vi "MACBIN Resource File Info Core__ogtk.vi"(5 "comment":string, 6 "error in (no error)":errorcluster, 7 "file info in":T1 {"mod date" format="%<%H:%M:%S\n%m/%d/%Y>T"; "creation date" format="%<%H:%M:%S\n%m/%d/%Y>T"}, 8 "write (F)":bool, 9 "resource file":path) -> (0 "error out":errorcluster, 1 "file info out":T1 {"mod date" format="%<%H:%M:%S\n%m/%d/%Y>T"; "creation date" format="%<%H:%M:%S\n%m/%d/%Y>T"}, 2 "is directory":bool, 3 "resource file out":path, 4 "comment out":string)   [LabVIEW 2014, in "ZLIB.lvlib"]
uses:
  ZLIB.lvlib
  MACBIN Resource Header__ogtk.ctl
  lvzlib.dll
panel:
  # "Please visit http://www.OpenG.org to learn about the\nOpen Source LabVIEW software movement.\n\nNOTICE -- YOU MUST LEAVE THIS NOTICE IN PLACE.  PER THE TERMS OF THE LICENSE BELOW, YOU MAY SUBLICENSE THIS SOFTWARE \nIN ANY WAY THAT DOES NOT CONFLICT WITH THIS LICENSE.\n\n### BSD License (http://www.opensource.org/licenses/bsd-license.php) Begin ###\n\nCopyright (C) 2006 Rolf Kalbermatter rolf.kalbermatter@citengineering.com\n\nAll rights reserved.\n\nRedistribution and use in source and binary forms, with or without modification, are permitted provided that the following conditions are met:\n\n    * Redistributions of source code must retain the above copyright notice, this list of conditions and the following disclaimer.\n    * Redistributions in binary form must reproduce the above copyright notice, this list of conditions and the following disclaimer in the \n       documentation and/or other materials provided with the distribution.\n    * Neither the name of SciWare, James Kring, Inc., nor the names of its contributors may be used to endorse or promote products derived \n       from this software without specific prior written permission.\n\nTHIS SOFTWARE IS PROVIDED BY THE COPYRIGHT HOLDERS AND CONTRIBUTORS \"AS IS\" AND ANY EXPRESS OR IMPLIED WARRANTIES, \nINCLUDING, BUT NOT LIMITED TO, THE IMPLIED WARRANTIES OF MERCHANTABILITY AND FITNESS FOR A PARTICULAR PURPOSE ARE \nDISCLAIMED. IN NO EVENT SHALL THE COPYRIGHT OWNER OR CONTRIBUTORS BE LIABLE FOR ANY DIRECT, INDIRECT, INCIDENTAL,\n SPECIAL, EXEMPLARY, OR CONSEQUENTIAL DAMAGES (INCLUDING, BUT NOT LIMITED TO, PROCUREMENT OF SUBSTITUTE GOODS OR \nSERVICES; LOSS OF USE, DATA, OR PROFITS; OR BUSINESS INTERRUPTION) HOWEVER CAUSED AND ON ANY THEORY OF LIABILITY, \nWHETHER IN CONTRACT, STRICT LIABILITY, OR TORT (INCLUDING NEGLIGENCE OR OTHERWISE) ARISING IN ANY WAY OUT OF THE USE \nOF THIS SOFTWARE, EVEN IF ADVISED OF THE POSSIBILITY OF SUCH DAMAGE.\n\n### BSD License End ###"
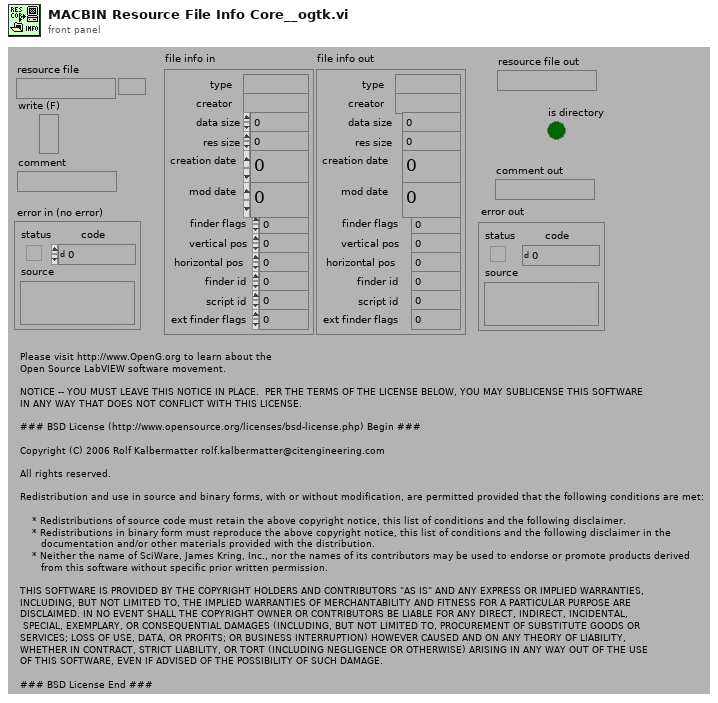
[diagram p1: front panel]
types:
  T1 = typedef "ZLIB.lvlib/MACBIN Resource Header__ogtk.ctl" = cluster{"type":string, "creator":string, "data size":u32, "res size":u32, "creation date":u32, "mod date":u32, "finder flags":u16, "vertical pos":i16, "horizontal pos":i16, "finder id":u16, "script id":u8, "ext finder flags":u8}
  T2 = cluster{"type":u32, "creator":u32, "data size":u32, "res size":u32, "creation date":u32, "mod date":u32, "finder flags":u16, "vertical pos":i16, "horizontal pos":i16, "finder id":u16, "script id":u8, "ext finder flags":u8}
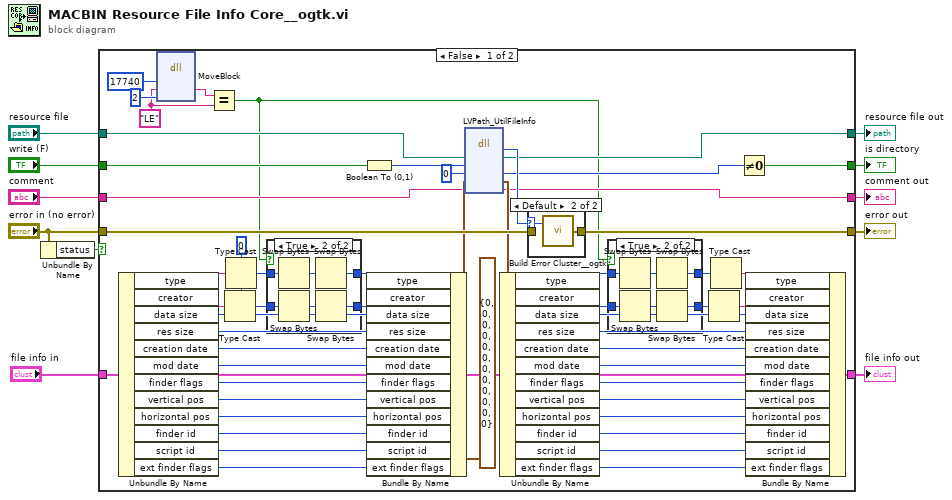
[diagram p0: block diagram]
diagram:
  n1 = Unbundle By Name("error in (no error)") -> ("status"=w2:bool)
  n2 = case shown="False" w2 {
    tunnel: [w27 w89] -> w7
    tunnel: "file info in" -> [w61 w90]
    tunnel: [w45 w90] -> w6
    tunnel: "comment" -> [w28 w89]
    tunnel: "write (F)" -> [w64 _]
    tunnel: [w65 w87] -> w9
    tunnel: "resource file" -> [w32 w88]
    tunnel: [w31 w88] -> w4
    tunnel: "error in (no error)" -> [w63 w87]
    tunnel: [w33 FALSE] -> w1
    frame False {
      w22 = "LE" ("y")
      w44 = u32 0 ("x")
      n3 = Unbundle By Name(w61) -> ("type"=w46:string, "creator"=w47:string, "data size"=w43:u32, "res size"=w42:u32, "creation date"=w41:u32, "mod date"=w40:u32, "finder flags"=w39:u16, "vertical pos"=w38:i16, "horizontal pos"=w37:i16, "finder id"=w36:u16, "script id"=w35:u8, "ext finder flags"=w34:u8)
      n4 = dll-call lib="LabVIEW" fn="MoveBlock"("src"=u16 17740, "dst"=w22, "len"=2) -> ("dst"=w21:string)  [unwired: 6 in, 2 out]
      n5 = Equal?(x=w21, y=w22) -> (x = y?=w12:bool)
      n6 = Type Cast(type=w44, x=w47) -> (*(type *) &x=w20:u32)
      n7 = Type Cast(type=w44, x=w46) -> (*(type *) &x=w19:u32)
      n8 = case shown="True" w12 {
        tunnel: w20 -> [w75 w82]
        tunnel: [w75 w80] -> w17
        tunnel: w19 -> [w76 w78]
        tunnel: [w76 w77] -> w18
        frame False {
        }
        frame True {
          n9 = Swap Bytes(anything=w78) -> (byte swapped=w79:u32)
          n10 = Swap Bytes(anything=w82) -> (byte swapped=w81:u32)
          n11 = Swap Bytes(anything=w79) -> (byte swapped=w77:u32)
          n12 = Swap Bytes(anything=w81) -> (byte swapped=w80:u32)
        }
      }
      n13 = Boolean To (0,1)(Boolean=w64) -> (0, 1=w62:i16)
      n14 = Bundle By Name(cluster=T2 {"type"=0, "creator"=0, "data size"=0, "res size"=0, "creation date"=0, "mod date"=0, "finder flags"=0, "vertical pos"=0, "horizontal pos"=0, "finder id"=0, "script id"=0, "ext finder flags"=0} ("file info in"), "type"=w18, "creator"=w17, "data size"=w43, "res size"=w42, "creation date"=w41, "mod date"=w40, "finder flags"=w39, "vertical pos"=w38, "horizontal pos"=w37, "finder id"=w36, "script id"=w35, "ext finder flags"=w34) -> (w30:T2)
      n15 = dll-call lib="C:/Users/Public/SSDC/OpenDocument/LabVIEWODFToolkit/Sourcecode/SubVIs/ZLIB/lvzlib.*" fn="LVPath_UtilFileInfo"("resource file"=w32, "write"=w62, "isDir"=u8 0, "file info in"=w30, "comment"=w28) -> (w66:i32, "resource file"=w31:path, "isDir"=w26:u8, "file info in"=w29:T2, "comment"=w27:string)  [unwired: 4 in, 2 out]
      n16 = Unbundle By Name(w29) -> ("type"=w13:u32, "creator"=w16:u32, "data size"=w57:u32, "res size"=w56:u32, "creation date"=w55:u32, "mod date"=w54:u32, "finder flags"=w53:u16, "vertical pos"=w52:i16, "horizontal pos"=w51:i16, "finder id"=w50:u16, "script id"=w49:u8, "ext finder flags"=w48:u8)
      n17 = case shown="Default" w66 {
        selector: w66 -> [_ w85]
        tunnel: [w83 w84] -> w65
        tunnel: w63 -> [w83 _]
        frame 0 {
        }
        frame Default {
          n18 = call "Build Error Cluster__ogtk.vi"("code"=w85) -> ("error out"=w84:errorcluster)  [unwired: 1 in]
        }
      }
      n19 = case shown="True" w12 {
        tunnel: w16 -> [w67 w74]
        tunnel: [w67 w72] -> w15
        tunnel: w13 -> [w68 w70]
        tunnel: [w68 w69] -> w14
        frame False {
        }
        frame True {
          n20 = Swap Bytes(anything=w70) -> (byte swapped=w71:u32)
          n21 = Swap Bytes(anything=w74) -> (byte swapped=w73:u32)
          n22 = Swap Bytes(anything=w71) -> (byte swapped=w69:u32)
          n23 = Swap Bytes(anything=w73) -> (byte swapped=w72:u32)
        }
      }
      n24 = Type Cast(x=w15) -> (*(type *) &x=w59:string)  [unwired: 1 in]
      n25 = Type Cast(x=w14) -> (*(type *) &x=w58:string)  [unwired: 1 in]
      n26 = Not Equal To 0?(x=w26) -> (x != 0?=w33:bool)
      n27 = Bundle By Name(cluster=w61, "type"=w58, "creator"=w59, "data size"=w57, "res size"=w56, "creation date"=w55, "mod date"=w54, "finder flags"=w53, "vertical pos"=w52, "horizontal pos"=w51, "finder id"=w50, "script id"=w49, "ext finder flags"=w48) -> (w45:T1)
    }
    frame True {
    }
  }
  "error out" <- w9
  "comment out" <- w7
  "file info out" <- w6
  "resource file out" <- w4
  "is directory" <- w1
